vi "Tosca-Count Frames.vi"(5 "StateDurs":dbl[](array[numeric]), 7 "FrameRate (Hz)":dbl, 9 "Index":i32=1, 11 "2P?":bool) -> (4 "Frames":i32)   [LabVIEW 2020]
uses:
  TTL VIs/Control Classes/Base Class/TTLController.lvclass
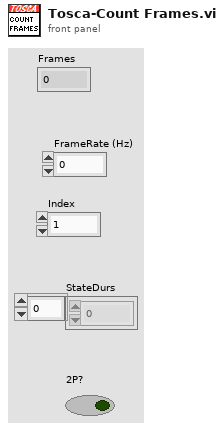
[diagram p1: front panel]
types:
  T1 = typedef "Tosca-Flow Element.ctl" = cluster{"Name":string, "State Index":i32, "Row":dbl, "Color":u32, "Selected?":bool, "Timeouts":T2[], "Term Cond":T4[], "rect":cluster{"left":i16, "top":i16, "right":i16, "bottom":i16}, "Target?":bool, "Links":cluster{"forward":i32[], "backward":i32[]}}
  T2 = typedef "Tosca-Timeout Spec.ctl" = cluster{"Next":i32, "rect":cluster{"left":i16, "top":i16, "right":i16, "bottom":i16}, "Row":dbl, "Selected?":bool, "Type":T3, "Units":enum16{"Reps", "Seconds"}, "Expr":string, "TTL":refnum<class "TTLController.lvclass">[]}
  T3 = typedef "Tosca-Event Type.ctl" = enum16{"Normal", "CS+", "CS-"}
  T4 = typedef "Tosca-Termination Condition.ctl" = cluster{"Name":string, "Input Event":i32, "Next":i32, "rect":cluster{"left":i16, "top":i16, "right":i16, "bottom":i16}, "Row":dbl, "Selected?":bool, "Type":T3, "End after (ms)":dbl, "End on rep":bool, "Latency (ms)":dbl, "TTL":refnum<class "TTLController.lvclass">[], "Action":T5, "Nttl":i32, "Tttl":string, "one shot":bool}
  T5 = typedef "Tosca-Termination Condition Action.ctl" = enum16{"End state", "Complete state", "TTL only"}
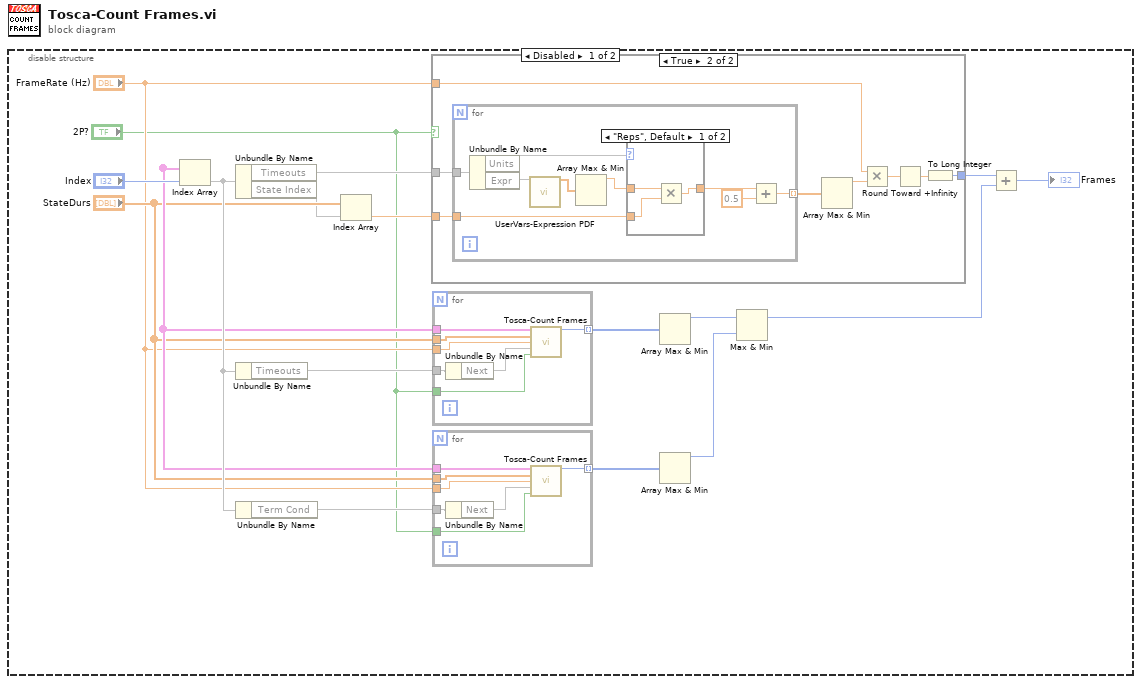
[diagram p0: block diagram]
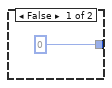
[diagram p2: hidden frame]
diagram:
  n1 = disable-structure shown="Disabled" {
    frame Disabled {
      n2 = Index Array(index="Index") -> (array=w9:T1[], element=w11)
      n3 = Unbundle By Name(w11) -> ("Timeouts"=w18, "State Index"=w6)
      n4 = Unbundle By Name(w11) -> ("Timeouts"=w15)
      n5 = Unbundle By Name(w11) -> ("Term Cond"=w10)
      n6 = Index Array(array="StateDurs", index=w6) -> (element=w16:dbl)
      n7 = case shown="True" "2P?" {
        tunnel: w18 -> [_ w41]
        tunnel: w16 -> [_ w40]
        tunnel: "FrameRate (Hz)" -> [_ w37]
        tunnel: [0 w34] -> w14
        frame False {
        }
        frame True {
          n8 = for {
            tunnel: w41 -> [w50]
            tunnel: w40 -> [w48]
            tunnel: [w45] -> w39 mode=indexing
            n9 = Unbundle By Name(w50) -> ("Units"=w49, "Expr"=w44)
            n10 = call "UserVars-Expression PDF.vi"("Expr"=w44) -> ("X"=w43:dbl[])  [unwired: 10 in, 4 out]
            n11 = Array Max & Min(array=w43) -> (max value=w42:dbl)  [unwired: 3 out]
            n12 = case shown="\"Reps\", Default" w49 {
              tunnel: [w52 w54] -> w47
              tunnel: w48 -> [w53 _]
              tunnel: w42 -> [w51 w54]
              frame "Reps", Default {
                n13 = Multiply(x=w51, y=w53) -> (x*y=w52:dbl)
              }
              frame "Seconds" {
              }
            }
            n14 = Add(x=w47, y=0.5) -> (x+y=w45:dbl)
          }
          n15 = Array Max & Min(array=w39) -> (max value=w38:dbl)  [unwired: 3 out]
          n16 = Multiply(x=w37, y=w38) -> (x*y=w36:dbl)
          n17 = Round Toward +Infinity(x=w36) -> (ceil(x): smallest int >= x=w35:dbl)
          n18 = To Long Integer(number=w35) -> (32bit integer=w34:i32)
        }
      }
      n19 = for {
        tunnel: w15 -> [w25]
        tunnel: [w23] -> w5 mode=indexing
        tunnel: w9 -> [w22]
        tunnel: "StateDurs" -> [w21]
        tunnel: "FrameRate (Hz)" -> [w20]
        tunnel: "2P?" -> [w19]
        n20 = Unbundle By Name(w25) -> ("Next"=w24)
        n21 = call "Tosca-Count Frames.vi"(0:w22, "StateDurs"=w21, "FrameRate (Hz)"=w20, "Index"=w24, "2P?"=w19) -> ("Frames"=w23:i32)  [unwired: 10 in]
      }
      n22 = for {
        tunnel: w10 -> [w32]
        tunnel: [w30] -> w4 mode=indexing
        tunnel: w9 -> [w29]
        tunnel: "StateDurs" -> [w28]
        tunnel: "FrameRate (Hz)" -> [w27]
        tunnel: "2P?" -> [w26]
        n23 = Unbundle By Name(w32) -> ("Next"=w31)
        n24 = call "Tosca-Count Frames.vi"(0:w29, "StateDurs"=w28, "FrameRate (Hz)"=w27, "Index"=w31, "2P?"=w26) -> ("Frames"=w30:i32)  [unwired: 10 in]
      }
      n25 = Array Max & Min(array=w5) -> (max value=w3:i32)  [unwired: 3 out]
      n26 = Array Max & Min(array=w4) -> (max value=w2:i32)  [unwired: 3 out]
      n27 = Max & Min(x=w3, y=w2) -> (max(x,y)=w12:i32)  [unwired: 1 out]
      n28 = Add(x=w14, y=w12) -> (x+y=→"Frames":i32)
    }
    frame Enabled {
    }
  }
